vi "Validate connection.vi"(8 "error in (no error)":errorcluster, 11 "VISA Refnum in":refnum<visa-resource-name>) -> (0 "error out":errorcluster, 2 "Connection valid?":bool, 3 "VISA Refnum out":refnum<visa-resource-name>)   [LabVIEW 2020, in "Arduino-Adafruit stepper.lvlib"]
uses:
  Arduino-Adafruit stepper.lvlib
  e00ded2c-1239-4006-9df9-6765111190f0.vi
  751c0b5a-9974-4f1b-8c00-a8daef4b7bb7.vi
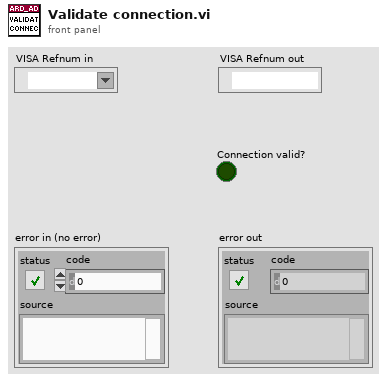
[diagram p1: front panel]
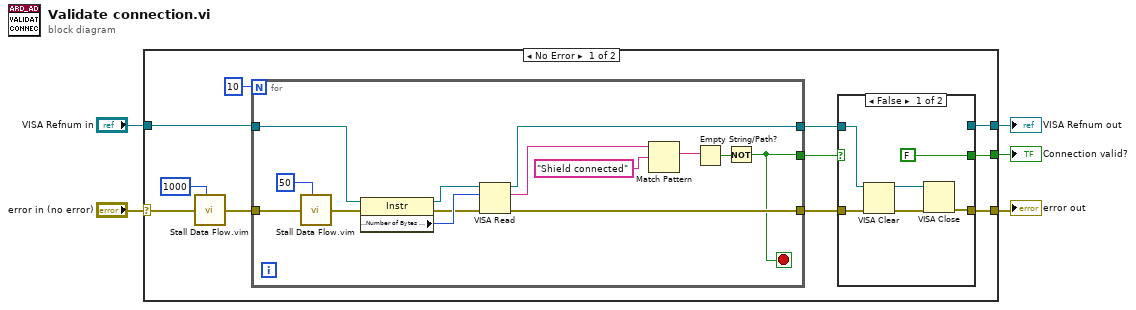
[diagram p0: block diagram]
diagram:
  n1 = case shown="No Error" "error in (no error)" {
    selector: "error in (no error)" -> [w15 w40]
    tunnel: "VISA Refnum in" -> [w16 w41]
    tunnel: [w10 w40] -> w3
    tunnel: [w7 _] -> w2
    tunnel: [w6 w41] -> w1
    frame No Error {
      n2 = call "Stall Data Flow.vim"("value in"=w15, "milliseconds to wait"=u32 1000) -> ("value out"=w12:errorcluster)  [unwired: 1 out]
      n3 = for {
        N: 10 -> [_]
        tunnel: [w39] -> w14
        tunnel: w16 -> [w30]
        tunnel: w12 -> [w28]
        tunnel: [w31] -> w8
        tunnel: [w26] -> w9
        stop <- w31 stop-if-true
        n4 = call "Stall Data Flow.vim"("value in"=w28, "milliseconds to wait"=u32 50) -> ("value out"=w27:errorcluster)  [unwired: 1 out]
        n5 = property class="Instr"(reference=w30, error in=w27) -> (reference out=w36:refnum<visa-resource-name>, error out=w37:errorcluster, "Serial Settings:Number of Bytes at Serial Port"=w38:u32)
        n6 = VISA Read(VISA resource name=w36, byte count=w38, error in (no error)=w37) -> (VISA resource name out=w26:refnum<visa-resource-name>, read buffer=w35:string, error out=w39:errorcluster)  [unwired: 1 out]
        n7 = Match Pattern(string=w35, regular expression="Shield connected") -> (match substring=w33:string)  [unwired: 1 in, 3 out]
        n8 = Empty String/Path?(string/path=w33) -> (empty?=w32:bool)
        n9 = Not(x=w32) -> (.not. x?=w31:bool)
      }
      n10 = case shown="False" w8 {
        selector: w8 -> [_ w24]
        tunnel: w14 -> [w22 w25]
        tunnel: [w18 w25] -> w10
        tunnel: w9 -> [w21 w23]
        tunnel: [FALSE w24] -> w7
        tunnel: [_ w23] -> w6
        frame False {
          n11 = VISA Clear(VISA resource name=w21, error in (no error)=w22) -> (VISA resource name out=w17:refnum<visa-resource-name>, error out=w19:errorcluster)
          n12 = VISA Close(VISA resource name=w17, error in (no error)=w19) -> (error out=w18:errorcluster)
        }
        frame True {
        }
      }
    }
    frame Error {
    }
  }
  "error out" <- w3
  "Connection valid?" <- w2
  "VISA Refnum out" <- w1
